vi "Test Not In Process Loop When Started.vi"(8 "error in (no error)":errorcluster, 11 "Test Case In":refnum<class "Process Lifecycle Test.lvclass">) -> (0 "error out":errorcluster, 3 "Test Case Out":refnum<class "Process Lifecycle Test.lvclass">)   [LabVIEW 2020, in "Process Lifecycle Test.lvclass"]
uses:
  Process Lifecycle Test.lvclass
  Process Lifecycle Test.lvclass/Process Lifecycle Test.ctl
  source/Framework/Process/Process.lvclass
  123a4b7f-48eb-4ca1-825a-3f73a8a1fba5.vi
  source/Framework/Process/Public/Lifecycle/API Mode.ctl
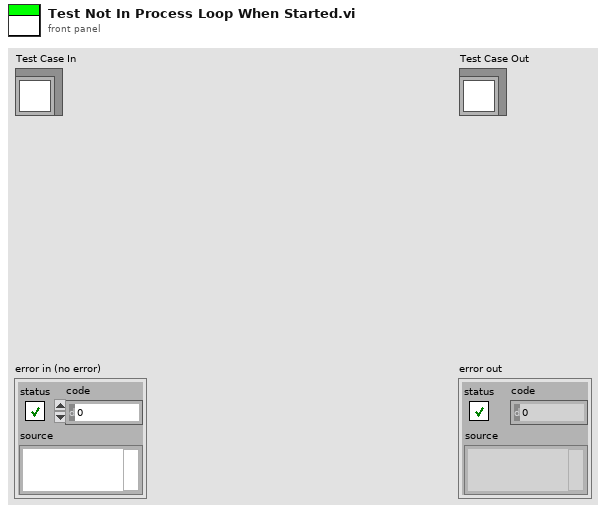
[diagram p1: front panel]
types:
  T1 = typedef "Process.lvclass/API Mode.ctl" = enum16{"Send Message", "Handle Message"}
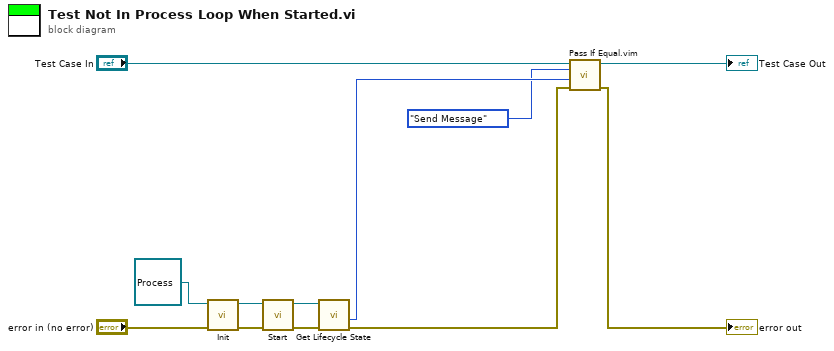
[diagram p0: block diagram]
diagram:
  n1 = call-dynamic "Init.vi"("error in (no error)"="error in (no error)", "Process In"=refnum<class "Process.lvclass"> refnum) -> ("error out"=w7:errorcluster, "Process Out"=w4:refnum<class "Process.lvclass">)  [unwired: 8 in]
  n2 = call "Start.vi"("error in (no error)"=w7, "Process In"=w4) -> ("error out"=w5:errorcluster, "Process Out"=w3:refnum<class "Process.lvclass">)  [unwired: 7 in, 1 out]
  n3 = call "Get Lifecycle State.vi"("error in (no error)"=w5, "Process In"=w3) -> ("error out"=w8:errorcluster, "API Mode"=w2:T1)  [unwired: 6 in, 2 out]
  n4 = call "Pass If Equal.vim"("error in (no error)"=w8, "Actual"=w2, "Expected"=API_Mode."Send Message" ("API Mode"), "LUnit Test Case In"="Test Case In") -> ("error out"=→"error out":errorcluster, "LUnit Test Case Out"=→"Test Case Out":refnum<class "Process Lifecycle Test.lvclass">)  [unwired: 6 in]
